vi "New Connection Handler.vi"(7 "Connection":refnum<class "IConnection.lvclass">, 8 "error in":errorcluster, 9 "Message Protocol":refnum<class "IMessagingProtocol.lvclass">, 10 "Controller Queue":refnum<class "Message Queue.lvclass">, 11 "Read Queue":refnum<queue>) -> (0 "error out":errorcluster, 3 "Handler Queue":refnum<class "Message Queue.lvclass">)   [LabVIEW 2017, in "Network Interface.lvlib" / "Connection Handler.lvclass"]
uses:
  <vilib>/gpm_packages/@cs/Network-sink/Source/Network Interface/Connection Handler/Connection Handler.lvclass
  <vilib>/gpm_packages/@cs/Network-sink/Source/Network Interface/IConnection/IConnection.lvclass
  <vilib>/gpm_packages/@cs/Network-sink/Source/Network Interface/IMessagingProtocol/IMessagingProtocol.lvclass
  <vilib>/gpm_packages/@cs/Network-sink/Source/Network Interface/Message Queue/Message Queue.lvclass
  <vilib>/gpm_packages/@cs/Network-sink/Source/Network Interface/Connection Handler/Connection Handler.lvclass/Connection Handler.ctl
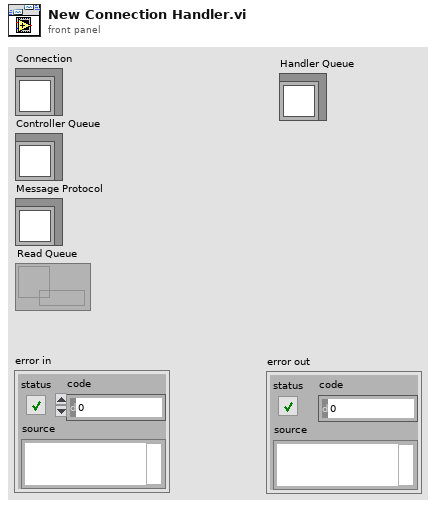
[diagram p1: front panel]
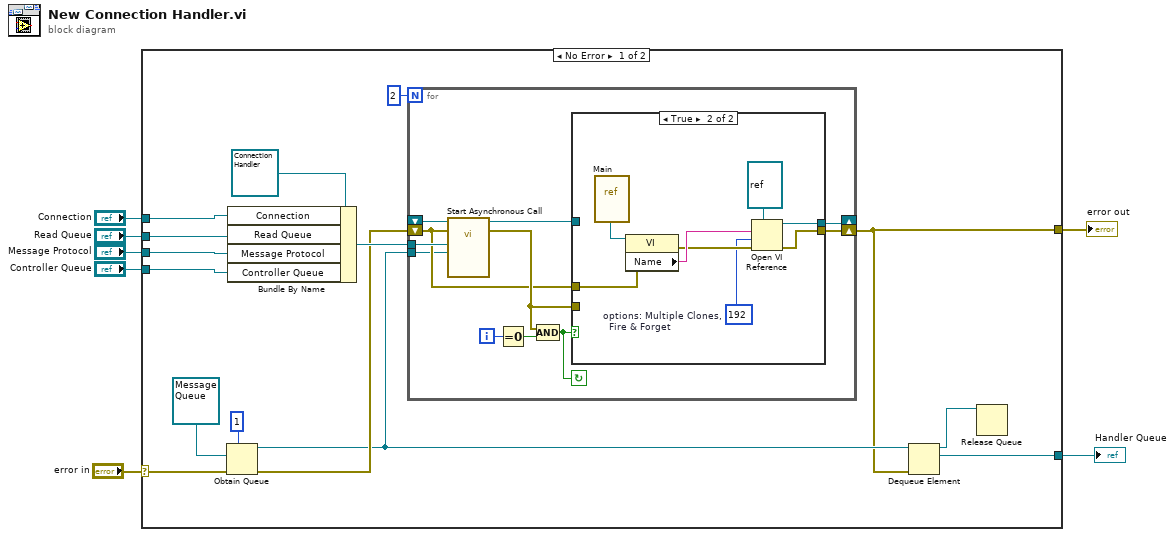
[diagram p0: block diagram]
diagram:
  n1 = case shown="No Error" "error in" {
    selector: "error in" -> [w14 w44]
    tunnel: "Connection" -> [w21 _]
    tunnel: "Read Queue" -> [w20 _]
    tunnel: "Message Protocol" -> [w19 _]
    tunnel: "Controller Queue" -> [w18 _]
    tunnel: [w10 w44] -> w2
    tunnel: [w9 _] -> w1
    frame No Error {
      n2 = Obtain Queue(max queue size (-1, unlimited)=1, element data type=refnum<class "Message Queue.lvclass"> refnum ("Controller Queue"), error in (no error)=w14) -> (queue out=w11:refnum<queue>, error out=w13:errorcluster)  [unwired: 2 in, 1 out]
      n3 = Bundle By Name(cluster=refnum<class "Connection Handler.lvclass"> refnum ("Connection Handler in"), "Connection"=w21, "Read Queue"=w20, "Message Protocol"=w19, "Controller Queue"=w18) -> (w17:refnum<class "Connection Handler.lvclass">)
      n4 = for {
        N: 2 -> [_]
        tunnel: w17 -> [w26]
        shift-right: [w32] -> _
        shift-left: _ -> [w33]
        shift-right: [w27] -> w10
        shift-left: w13 -> [w25]
        tunnel: w11 -> [w24]
        i -> [w29]
        stop <- w23 continue-if-true
        n5 = call-by-ref "Start Asynchronous Call"(reference=w33, error in=w25, "Caller Return Queue"=w24, "Connection Handler in"=w26) -> (reference out=w31:refnum<vi>, error out=w28:errorcluster)  [unwired: 10 in]
        n6 = Equal To 0?(x=w29) -> (x = 0?=w30:bool)
        n7 = Compound Arithmetic op=AND(w28, w30) -> (w23:bool)
        n8 = case shown="True" w23 {
          tunnel: [w35 w40] -> w32
          tunnel: w31 -> [w35 _]
          tunnel: w28 -> [w34 _]
          tunnel: [w34 w38] -> w27
          tunnel: w25 -> [_ w37]
          frame False {
          }
          frame True {
            w36 = 192  # options: Multiple Clones,   Fire & Forget
            n9 = vi-ref <vilib>:"Main.vi"() -> (w43:refnum<vi>)
            n10 = property class="VI"(reference=w43, error in=w37) -> (error out=w39:errorcluster, "Name"=w42:string)  [unwired: 1 out]
            n11 = Open VI Reference(type specifier VI Refnum (for type only)=refnum<vi> refnum, vi path=w42, options=w36, error in (no error)=w39) -> (vi reference=w40:refnum<vi>, error out=w38:errorcluster)  [unwired: 2 in]
          }
        }
      }
      n12 = Dequeue Element(queue=w11, error in (no error)=w10) -> (queue out=w8:refnum<queue>, element=w9:refnum<class "Message Queue.lvclass">)  [unwired: 1 in, 2 out]
      n13 = Release Queue(queue=w8) -> ()  [unwired: 2 in, 3 out]
    }
    frame Error {
    }
  }
  "error out" <- w2
  "Handler Queue" <- w1
